vi "Error Cluster From Error Status Bit.vi"(8 "error in (no error)":errorcluster, 10 "Error Status Bit (Command Error)":T1=7 items=["Counter Overrun"=3, "Rate Error"=4, "Recall Error"=5, "Command Error"=7], 11 "VISA resource name":refnum<visa-resource-name>) -> (0 "error out":errorcluster, 3 "VISA resource name out":refnum<visa-resource-name>)   [LabVIEW 2015, in "SRS SR400.lvlib"]
doc: "Reads the error status bit wired to the Error Status Bit terminal using the <B>SS</B> command, and generates an error cluster if the bit is enabled.\n\nThe SR400 has four error status bits:\n\n<B>Bit</B> <B>Error</B>\n3 Counter Overrun\n4 Rate Error\n5 Recall Error\n7 Command Error"
uses:
  SRS SR400.lvlib
  Typedefs/Error Codes Matrix.ctl
  Typedefs/Error Status Bit.ctl
panel:
  in  "Error Codes Matrix":T2=[["", ""], ["", ""], ["", ""], ["3", "Counter Overrun. This bit is set whenever counter A or B exceeds or equals 10^9 - 1 counts."], ["4", "Rate Error. This bit is set whenever a gate is missed. This can occur if a gate delay or width exceeds the trigger period minus 1 µs."], ["5", "Recall Error. This bit is set if a recall from a stored setting detects an error in the recalled data. If an error is found, the instrument setup is not altered."], ["", ""], ["7", "Command Error. This bit is set when an illegal command is received."]]
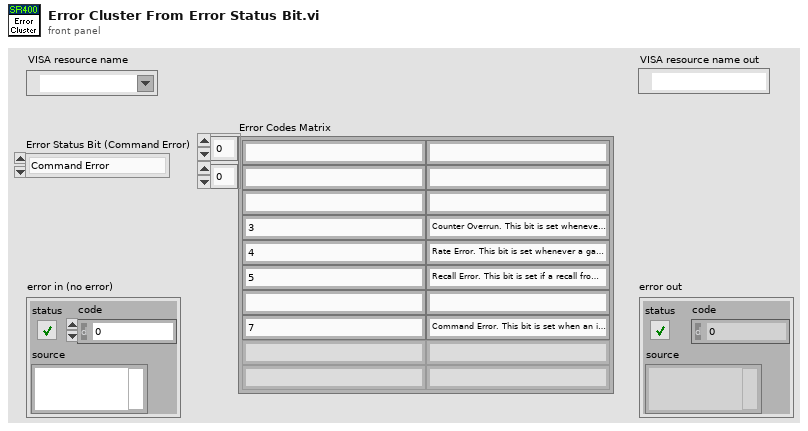
[diagram p1: front panel]
types:
  T1 = typedef "SRS SR400.lvlib/Error Status Bit.ctl" = u16
  T2 = typedef "SRS SR400.lvlib/Error Codes Matrix.ctl" = string[][]
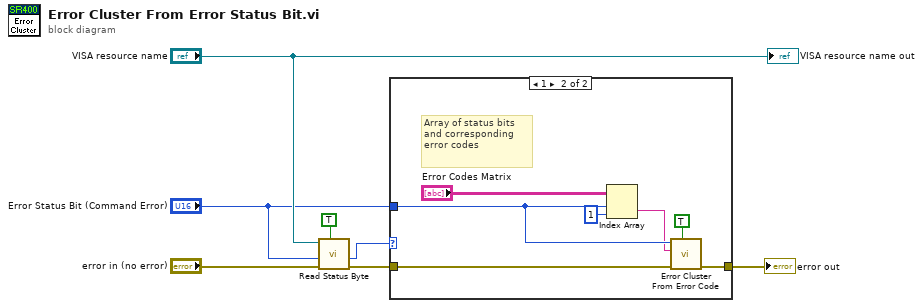
[diagram p0: block diagram]
diagram:
  n1 = call "Read Status Byte.vi"("Read Status Bit? (F)"=TRUE, "error in (no error)"="error in (no error)", "Status Bit (Scan Finished)"="Error Status Bit (Command Error)", "VISA resource name"="VISA resource name") -> ("error out"=w6:errorcluster, "Status Bit"=w5:u8)  [unwired: 4 in, 2 out]
  n2 = case shown="1" w5 {
    tunnel: w6 -> [w8 w15]
    tunnel: [w8 w14] -> w7
    tunnel: "Error Status Bit (Command Error)" -> [_ w11]
    frame 0, Default {
    }
    frame 1 {
      # "Array of status bits and corresponding error codes"
      n3 = Index Array(array="Error Codes Matrix", index (row)=w11, index (col)=1 ("disabled index (col)")) -> (element=w9:string)
      n4 = call <vilib>:"Error Cluster From Error Code.vi"("show call chain? (False)"=TRUE, "error in (no error)"=w15, "error message (\"\")"=w9, "error code (0)"=w11) -> ("error out"=w14:errorcluster)  [unwired: 5 in]
    }
  }
  "error out" <- w7
  "VISA resource name out" <- "VISA resource name"
